vi "Get Crafting Stations.vi"(8 "error in (no error)":errorcluster, 11 "Metal in":refnum<class "Metal.lvclass">) -> (0 "error out":errorcluster, 2 "Stations":T1[](array[typedef]), 3 "Metal out":refnum<class "Metal.lvclass">)   [LabVIEW 2020, in "Metal.lvclass"]
uses:
  Metal.lvclass
  Item/Craft Station.ctl
  Workstation/Workstation.lvclass
  Item/Item.lvclass
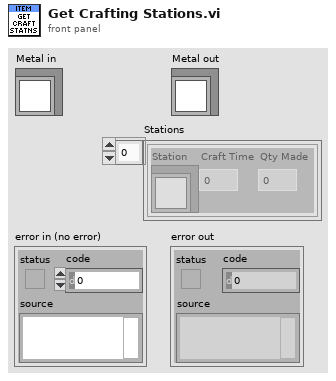
[diagram p1: front panel]
types:
  T1 = typedef "Item.lvclass/Craft Station.ctl" = cluster{"Station":refnum<class "Workstation.lvclass">, "Craft Time":dbl, "Qty Made":dbl}
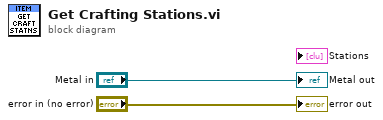
[diagram p0: block diagram]
diagram:
  "error out" <- "error in (no error)"
  "Metal out" <- "Metal in"
